vi "_AllThingsBS.vi"   [LabVIEW 2012]
uses:
  <userlib>/botspeak/VIs/BotSpeak.lvclass
  <vilib>/NXT/LegoClasses/BrickManagers/BotSpeakManager/BotSpeakManager.lvclass
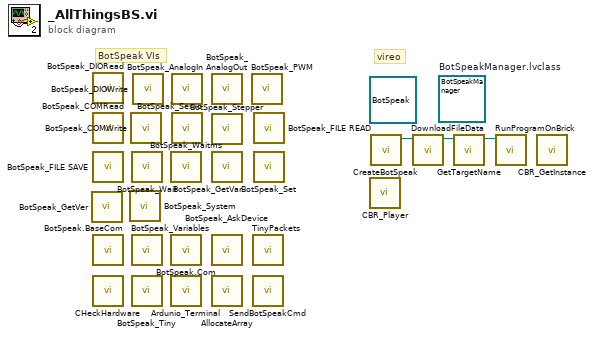
[diagram p0: block diagram]
diagram:
  (unwired) refnum<class "BotSpeakManager.lvclass"> refnum  # BotSpeakManager.lvclass
  (unwired) refnum<class "BotSpeak.lvclass"> refnum ("BotSpeak.lvclass")
  # "vireo"
  # "BotSpeak VIs"
  n1 = call <userlib>:"BotSpeak_GetVer.vi"() -> ()  [unwired: 2 in, 2 out]
  n2 = call <userlib>:"BotSpeak_DIORead.vi"() -> ()  [unwired: 3 in, 2 out]
  n3 = call <userlib>:"BotSpeak_COMRead.vi"() -> ()  [unwired: 3 in, 2 out]
  n4 = call <userlib>:"BotSpeak_FILE SAVE.vi"() -> ()  [unwired: 4 in, 1 out]
  n5 = call <userlib>:"BotSpeak.BaseCom.vi"() -> ()  [unwired: 5 in, 2 out]
  n6 = call <userlib>:"CHeckHardware.vi"() -> ()  [unwired: 3 in, 1 out]
  n7 = call <userlib>:"BotSpeak_System.vi"() -> ()  [unwired: 4 in, 1 out]
  n8 = call <userlib>:"BotSpeak_COMWrite.vi"() -> ()  [unwired: 3 in, 2 out]
  n9 = call <userlib>:"BotSpeak_Wait.vi"() -> ()  [unwired: 3 in, 1 out]
  n10 = call <userlib>:"BotSpeak_Variables.vi"() -> ()  [unwired: 3 in, 1 out]
  n11 = call <userlib>:"BotSpeak_Tiny.vi"() -> ()  [unwired: 2 in, 3 out]
  n12 = call <userlib>:"BotSpeak_DIOWrite.vi"() -> ()  [unwired: 4 in, 1 out]
  n13 = call <userlib>:"BotSpeak_Waitms.vi"() -> ()  [unwired: 3 in, 1 out]
  n14 = call <userlib>:"BotSpeak.Com.vi"() -> ()  [unwired: 3 in, 4 out]
  n15 = call <userlib>:"Ardunio_Terminal.vi"() -> ()  [unwired: 12 in]
  n16 = call <userlib>:"BotSpeak_AnalogIn.vi"() -> ()  [unwired: 3 in, 2 out]
  n17 = call <userlib>:"BotSpeak_Servo.vi"() -> ()  [unwired: 4 in, 1 out]
  n18 = call <userlib>:"BotSpeak_AnalogOut.vi"() -> ()  [unwired: 4 in, 1 out]
  n19 = call <userlib>:"BotSpeak_Stepper.vi"() -> ()  [unwired: 4 in, 1 out]
  n20 = call <userlib>:"BotSpeak_GetVar.vi"() -> ()  [unwired: 2 in, 2 out]
  n21 = call <userlib>:"BotSpeak_AskDevice.vi"() -> ()  [unwired: 3 in, 1 out]
  n22 = call <userlib>:"AllocateArray.vi"() -> ()  [unwired: 3 in, 1 out]
  n23 = call <userlib>:"BotSpeak_PWM.vi"() -> ()  [unwired: 4 in, 1 out]
  n24 = call <userlib>:"TinyPackets.vi"() -> ()  [unwired: 4 in, 1 out]
  n25 = call <userlib>:"SendBotSpeakCmd.vi"() -> ()  [unwired: 4 in, 2 out]
  n26 = call <userlib>:"BotSpeak_FILE READ.vi"() -> ()  [unwired: 3 in, 2 out]
  n27 = call <userlib>:"BotSpeak_Set.vi"() -> ()  [unwired: 4 in, 1 out]
  n28 = call <userlib>:"CBR_Player.vi"() -> ()  [unwired: 12 in]
  n29 = call <userlib>:"CreateBotSpeak.vi"() -> ("VIA.lvclass"=w3:refnum<class "BotSpeak.lvclass">)  [unwired: 11 in]
  n30 = call-dynamic "DownloadFileData.vi"("VIA in"=w3) -> ("VIA out"=w2:refnum<class "BotSpeak.lvclass">)  [unwired: 7 in, 3 out]
  n31 = call-dynamic "GetTargetName.vi"("VIA in"=w2) -> ("VIA out"=w1:refnum<class "BotSpeak.lvclass">)  [unwired: 8 in, 2 out]
  n32 = call-dynamic "RunProgramOnBrick.vi"("VIA in"=w1) -> ()  [unwired: 9 in, 2 out]
  n33 = call <userlib>:"CBR_GetInstance.vi"() -> ()  [unwired: 3 in, 1 out]
